vi "AssembleSiPCB - Copy.vi"() -> ()   [LabVIEW 2019]
panel:
  in  "VacCheck":bool
  in  "BPU":dbl
  in  "PCBU":dbl
  in  "SiU":dbl
  in  "U_Tool":dbl=90.0
  in  "SiAssemblyVacs":u64[](array[numeric])=[2097216, 2162754, 35717186, 52428866, 2098242]
  in  "PCBAssemblyVacs":u64[](array[numeric])=[4194368, 4456514, 38010946, 54526018, 4195394]
  in  "BPZ":dbl
  in  "BPY":dbl=882.875
  in  "BPX":dbl=250.748
  in  "GoToBP":bool
  in  "PickSiPCB":bool
  in  "PCBY":dbl=876.2095
  in  "PCBZ":dbl
  in  "PCBX":dbl=1126.3618
  in  "AssmbType":enum16{"Sensor", "PCB"}(ring)
  in  "SiY":dbl=876.3525
  in  "SiZ":dbl
  in  "SiX":dbl=824.1319
  in  "GoToSenPCB":bool
  in  "DropTool":bool
  in  "PickTool":bool
  in  "GoToToolPos":bool
  in  "X":dbl=548.9198 format="%#_7g"
  in  "Y":dbl=876.47257 format="%#_7g"
  in  "Z":dbl
  # "ToolPosition1"
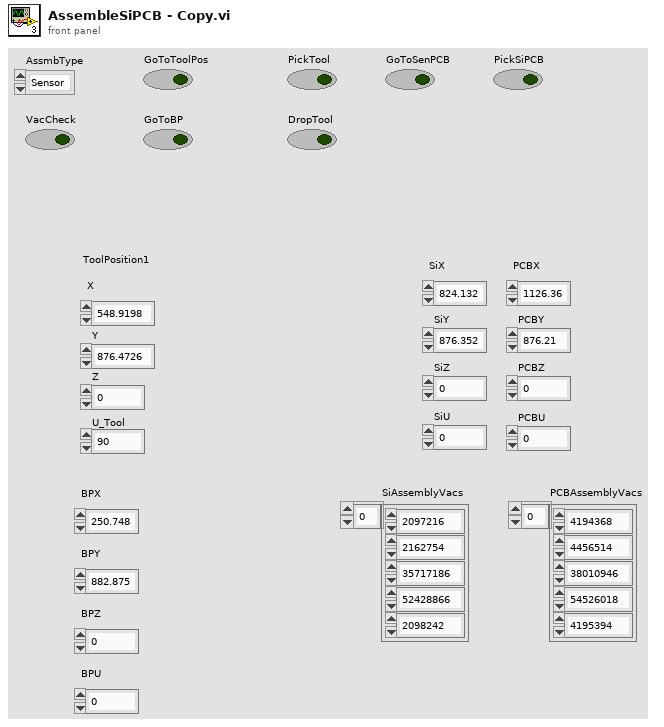
[diagram p1: front panel]
types:
  T1 = enum16{"Conversion", "BinarySwitch", "DecimalSwitch"}
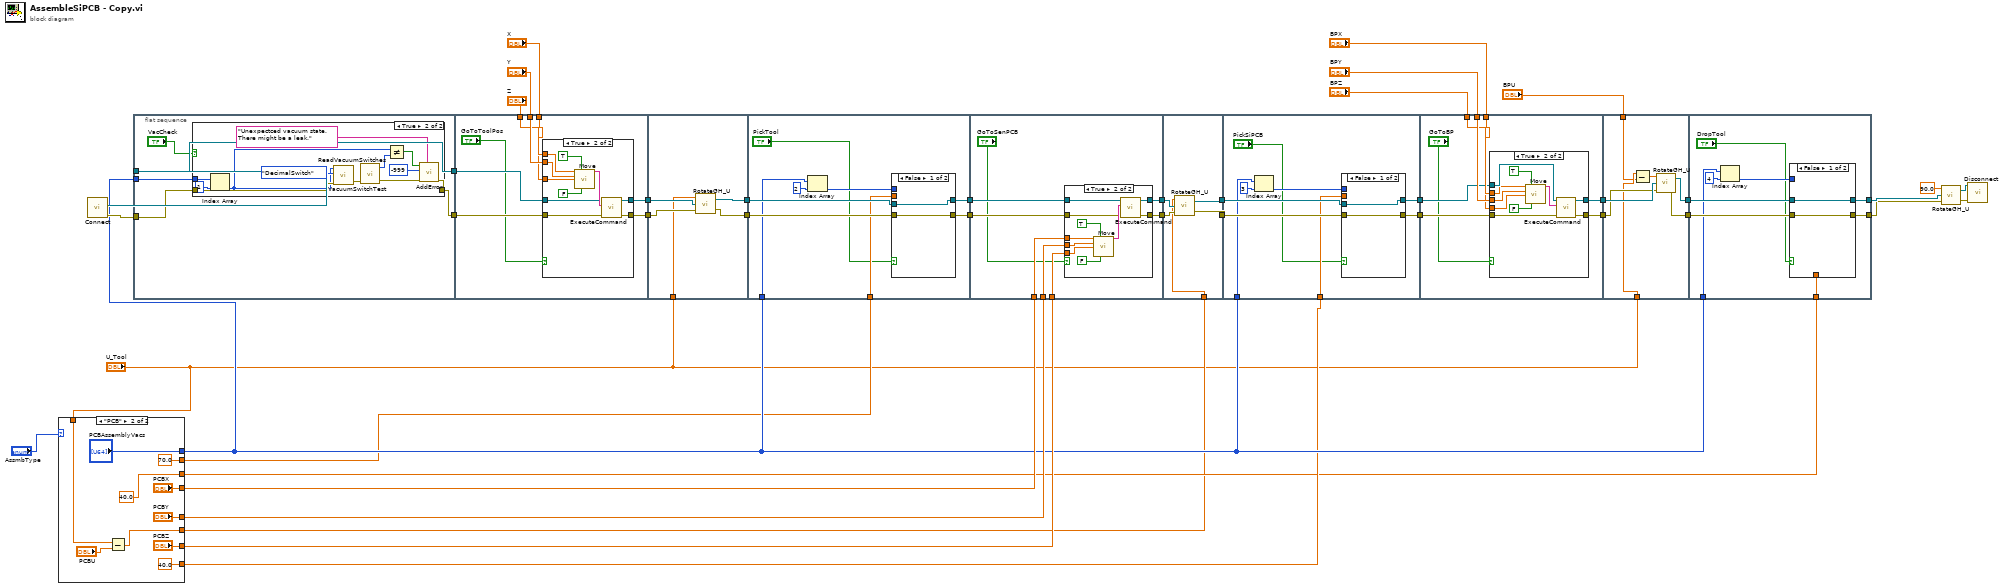
[diagram p0: block diagram]
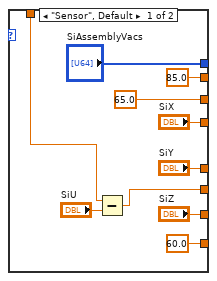
[diagram p2: hidden frame]
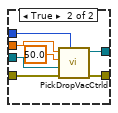
[diagram p5: hidden frame]
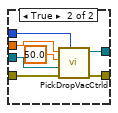
[diagram p7: hidden frame]
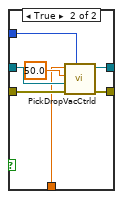
[diagram p9: hidden frame]
diagram:
  n1 = case shown="\"PCB\"" "AssmbType" {
    tunnel: ["SiX" "PCBX"] -> w32
    tunnel: ["SiY" "PCBY"] -> w31
    tunnel: ["SiZ" "PCBZ"] -> w30
    tunnel: ["SiAssemblyVacs" "PCBAssemblyVacs"] -> w24
    tunnel: [85.0 ("Z") 70.0 ("Z")] -> w23
    tunnel: [60.0 ("Z") 40.0 ("Z")] -> w22
    tunnel: [65.0 ("Z") 40.0 ("Z")] -> w21
    tunnel: "U_Tool" -> [w44 w54]
    tunnel: [w43 w53] -> w12
    frame "Sensor", Default {
      n2 = Subtract(x=w44, y="SiU") -> (x-y=w43:dbl)
    }
    frame "PCB" {
      n3 = Subtract(x=w54, y="PCBU") -> (x-y=w53:dbl)
    }
  }
  n4 = call "Connect.vi"() -> ("error out"=w41:errorcluster, "controller"=w42:refnum<k24>)  [unwired: 10 in]
  n5 = flat-sequence {
    tunnel: w41 -> [w67]
    tunnel: w42 -> [w66]
    tunnel: [w66] -> w37
    tunnel: [w64] -> w36
    tunnel: w24 -> [w65]
    tunnel: "X" -> [w86]
    tunnel: "Y" -> [w85]
    tunnel: "Z" -> [w84]
    tunnel: w37 -> [w88]
    tunnel: w36 -> [w87]
    tunnel: [w83] -> w20
    tunnel: [w82] -> w18
    tunnel: w20 -> [w105]
    tunnel: [w104] -> w19
    tunnel: w18 -> [w103]
    tunnel: [w102] -> w17
    tunnel: "U_Tool" -> [w101]
    tunnel: w19 -> [w114]
    tunnel: w17 -> [w113]
    tunnel: [w112] -> w35
    tunnel: [w111] -> w34
    tunnel: w24 -> [w108]
    tunnel: w23 -> [w107]
    tunnel: w35 -> [w128]
    tunnel: [w129] -> w16
    tunnel: w34 -> [w130]
    tunnel: [w131] -> w14
    tunnel: w32 -> [w127]
    tunnel: w31 -> [w126]
    tunnel: w30 -> [w125]
    tunnel: w16 -> [w148]
    tunnel: [w145] -> w15
    tunnel: w14 -> [w147]
    tunnel: [w146] -> w13
    tunnel: w12 -> [w144]
    tunnel: w15 -> [w156]
    tunnel: w13 -> [w157]
    tunnel: [w155] -> w29
    tunnel: [w154] -> w28
    tunnel: w24 -> [w151]
    tunnel: w22 -> [w150]
    tunnel: w29 -> [w171]
    tunnel: [w168] -> w11
    tunnel: w28 -> [w170]
    tunnel: [w169] -> w9
    tunnel: "BPX" -> [w174]
    tunnel: "BPY" -> [w173]
    tunnel: "BPZ" -> [w172]
    tunnel: w11 -> [w192]
    tunnel: [w191] -> w10
    tunnel: w9 -> [w193]
    tunnel: [w190] -> w8
    tunnel: "U_Tool" -> [w188]
    tunnel: "BPU" -> [w187]
    tunnel: [w199] -> w5
    tunnel: w10 -> [w201]
    tunnel: [w200] -> w4
    tunnel: w24 -> [w197]
    tunnel: w21 -> [w195]
    tunnel: w8 -> [w202]
    frame #0 {
      n6 = case shown="True" "VacCheck" {
        tunnel: w67 -> [w68 w79]
        tunnel: w65 -> [_ w78]
        tunnel: [w68 w72] -> w64
        frame False {
        }
        frame True {
          n7 = Index Array(array=w78, index=1) -> (element=w75:u64)
          n8 = call "VacuumSwitchTest.vi"("error in"=w79, "ControlType"=T1."DecimalSwitch", "DecimalIn"=w75) -> ("error out"=w76:errorcluster)  [unwired: 1 in, 2 out]
          n9 = call "ReadVacuumSwitches.vi"("error in"=w76) -> ("OutVacStatus"=w74:u32, "error out"=w73:errorcluster)  [unwired: 4 in, 1 out]
          n10 = Not Equal?(x=w75, y=w74) -> (x != y?=w70:bool)
          n11 = call "AddError.vi"("ErrorMessage"="Unexpectced vacuum state. There might be a leak.", "error in"=w73, "code"=-999, "Error?"=w70) -> ("Error out"=w72:errorcluster)  [unwired: 7 in]
        }
      }
    }
    frame #1 {
      n12 = case shown="True" "GoToToolPos" {
        tunnel: w88 -> [w90 w97]
        tunnel: w87 -> [w89 w96]
        tunnel: [w89 w95] -> w82
        tunnel: [w90 w94] -> w83
        tunnel: w86 -> [_ w93]
        tunnel: w85 -> [_ w92]
        tunnel: w84 -> [_ w91]
        frame False {
        }
        frame True {
          n13 = call "Move.vi"("X"=w93, "Absolute"=TRUE, "Y"=w92, "Z"=w91, "Move Z first"=FALSE) -> ("Position Gcode"=w98:string)  [unwired: 10 in]
          n14 = call "ExecuteCommand.vi"("error in (no error)"=w96, "Command Code"=w98, "controller in"=w97) -> ("error out"=w95:errorcluster, "controller out"=w94:refnum<k24>)  [unwired: 6 in, 1 out]
        }
      }
    }
    frame #2 {
      n15 = call "RotateGH_U.vi"("error in (no error)"=w103, "controller in"=w105, "U"=w101) -> ("error out"=w102:errorcluster, "controller out"=w104:refnum<k24>)
    }
    frame #3 {
      n16 = Index Array(array=w108, index=2) -> (element=w109:u64)
      n17 = case shown="False" "PickTool" {
        tunnel: w114 -> [w116 w122]
        tunnel: w113 -> [w115 w121]
        tunnel: w109 -> [_ w120]
        tunnel: [w116 w119] -> w112
        tunnel: [w115 w118] -> w111
        tunnel: w107 -> [_ w117]
        frame False {
        }
        frame True {
          n18 = call "PickDropVacCtrld.vi"("VacuumState"=w120, "error in (no error)"=w121, "controller in"=w122, "Zspeed"=50.0, "Z"=w117) -> ("error out"=w118:errorcluster, "controller out"=w119:refnum<k24>)  [unwired: 5 in]
        }
      }
    }
    frame #4 {
      n19 = case shown="True" "GoToSenPCB" {
        tunnel: [w133 w134] -> w131
        tunnel: w130 -> [w133 w136]
        tunnel: [w132 w135] -> w129
        tunnel: w128 -> [w132 w137]
        tunnel: w127 -> [_ w140]
        tunnel: w126 -> [_ w139]
        tunnel: w125 -> [_ w138]
        frame False {
        }
        frame True {
          n20 = call "Move.vi"("X"=w140, "Absolute"=TRUE, "Y"=w139, "Z"=w138, "Move Z first"=FALSE) -> ("Position Gcode"=w141:string)  [unwired: 10 in]
          n21 = call "ExecuteCommand.vi"("error in (no error)"=w136, "Command Code"=w141, "controller in"=w137) -> ("error out"=w134:errorcluster, "controller out"=w135:refnum<k24>)  [unwired: 6 in, 1 out]
        }
      }
    }
    frame #5 {
      n22 = call "RotateGH_U.vi"("error in (no error)"=w147, "controller in"=w148, "U"=w144) -> ("error out"=w146:errorcluster, "controller out"=w145:refnum<k24>)
    }
    frame #6 {
      n23 = Index Array(array=w151, index=3) -> (element=w152:u64)
      n24 = case shown="False" "PickSiPCB" {
        tunnel: w156 -> [w159 w165]
        tunnel: w157 -> [w158 w164]
        tunnel: [w159 w163] -> w154
        tunnel: [w158 w162] -> w155
        tunnel: w152 -> [_ w161]
        tunnel: w150 -> [_ w160]
        frame False {
        }
        frame True {
          n25 = call "PickDropVacCtrld.vi"("VacuumState"=w161, "error in (no error)"=w164, "controller in"=w165, "Zspeed"=50.0, "Z"=w160) -> ("error out"=w162:errorcluster, "controller out"=w163:refnum<k24>)  [unwired: 5 in]
        }
      }
    }
    frame #7 {
      n26 = case shown="True" "GoToBP" {
        tunnel: [w176 w180] -> w168
        tunnel: w171 -> [w176 w182]
        tunnel: [w175 w181] -> w169
        tunnel: w170 -> [w175 w183]
        tunnel: w174 -> [_ w179]
        tunnel: w173 -> [_ w178]
        tunnel: w172 -> [_ w177]
        frame False {
        }
        frame True {
          n27 = call "Move.vi"("X"=w179, "Absolute"=TRUE, "Y"=w178, "Z"=w177, "Move Z first"=FALSE) -> ("Position Gcode"=w184:string)  [unwired: 10 in]
          n28 = call "ExecuteCommand.vi"("error in (no error)"=w182, "Command Code"=w184, "controller in"=w183) -> ("error out"=w180:errorcluster, "controller out"=w181:refnum<k24>)  [unwired: 6 in, 1 out]
        }
      }
    }
    frame #8 {
      n29 = Subtract(x=w188, y=w187) -> (x-y=w189:dbl)
      n30 = call "RotateGH_U.vi"("error in (no error)"=w192, "controller in"=w193, "U"=w189) -> ("error out"=w191:errorcluster, "controller out"=w190:refnum<k24>)
    }
    frame #9 {
      n31 = Index Array(array=w197, index=4) -> (element=w196:u64)
      n32 = case shown="False" "DropTool" {
        tunnel: w202 -> [w204 w210]
        tunnel: w201 -> [w203 w209]
        tunnel: [w204 w208] -> w199
        tunnel: [w203 w207] -> w200
        tunnel: w196 -> [_ w206]
        tunnel: w195 -> [_ w205]
        frame False {
        }
        frame True {
          n33 = call "PickDropVacCtrld.vi"("VacuumState"=w206, "error in (no error)"=w209, "controller in"=w210, "Zspeed"=50.0, "Z"=w205) -> ("error out"=w207:errorcluster, "controller out"=w208:refnum<k24>)  [unwired: 5 in]
        }
      }
    }
  }
  n34 = call "RotateGH_U.vi"("error in (no error)"=w4, "controller in"=w5, "U"=90.0) -> ("error out"=w3:errorcluster, "controller out"=w2:refnum<k24>)
  n35 = call "Disconnect.vi"("error in (no error)"=w3, "controller"=w2) -> ()  [unwired: 9 in, 1 out]
